vi "Test-DotNet-Event.vi"() -> ()   [LabVIEW 2013, in "EC1000-control.lvlib" / "SM1000-control.lvclass"]
uses:
  SM1000-control.lvclass
  EC1000_DOTNET/getBroadcastData-status.vi
  C:/Users/vangeste/Desktop/Libraries/EC1000-control/LECSession.dll
  LECSession.dll
  Device-identification.ctl
  DOTNET-settings.ctl
  Fixed-data-type.ctl
  Status-information.ctl
panel:
  out "serverList iterator":i32
  out "Status information":T1
  out "Job count":i32
  out "Job name list":string
  out "Fixed data":string
  in  "File name wo extension":string="AdminConfig"
  in  "Fixed data type":T2=10 items=["Controller Configuration"=5, "Laser Configuration"=6, "Lens Configuration"=2, "Correction Table"=13, "User Configuration"=15, "Performance Adjustments"=16, "Admin Configuration"=10]
  in  "Device index":i32
  out "piServerCount":i32
  out "Device identifiers":T3[](array[typedef])
  in  "DOTNET settings":T4={"Target IP"="128.178.146.163", "Target broadcast port"=11000, "Target communication port"=12200, "clientID"=-1, "Broadcast IP"="224.168.100.2", "Servercount"=-1, "Device IDs"=[]}
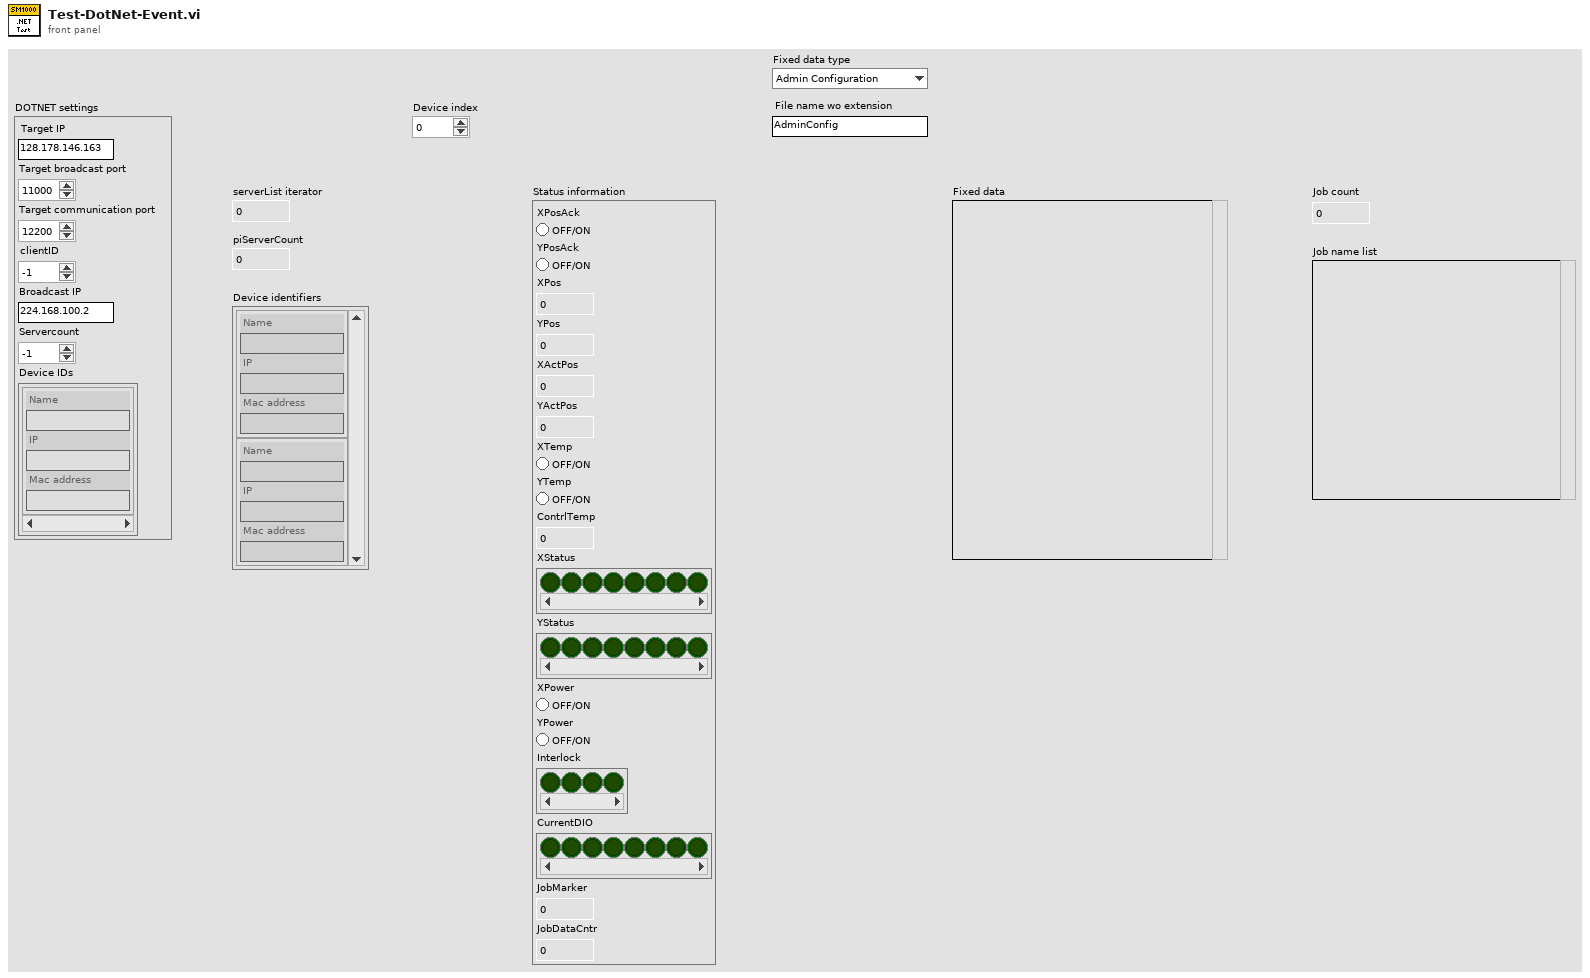
[diagram p1: front panel]
types:
  T1 = typedef "EC1000-control.lvlib/SM1000-control.lvclass/Status-information.ctl" = cluster{"XPosAck":bool, "YPosAck":bool, "XPos":i16, "YPos":i16, "XActPos":i16, "YActPos":i16, "XTemp":bool, "YTemp":bool, "ContrlTemp":i16, "XStatus":bool[], "YStatus":bool[], "XPower":bool, "YPower":bool, "Interlock":bool[], "CurrentDIO":bool[], "JobMarker":u16, "JobDataCntr":u32}
  T2 = typedef "EC1000-control.lvlib/SM1000-control.lvclass/Fixed-data-type.ctl" = i32
  T3 = typedef "EC1000-control.lvlib/SM1000-control.lvclass/Device-identification.ctl" = cluster{"Name":string, "IP":string, "Mac address":string}
  T4 = typedef "EC1000-control.lvlib/SM1000-control.lvclass/DOTNET-settings.ctl" = cluster{"Target IP":string, "Target broadcast port":i32, "Target communication port":i32, "clientID":i32, "Broadcast IP":string, "Servercount":i32, "Device IDs":T3[]}
  T5 = typedef "EC1000-control.lvlib/SM1000-control.lvclass/Object-reference.ctl" = refnum<data-value>
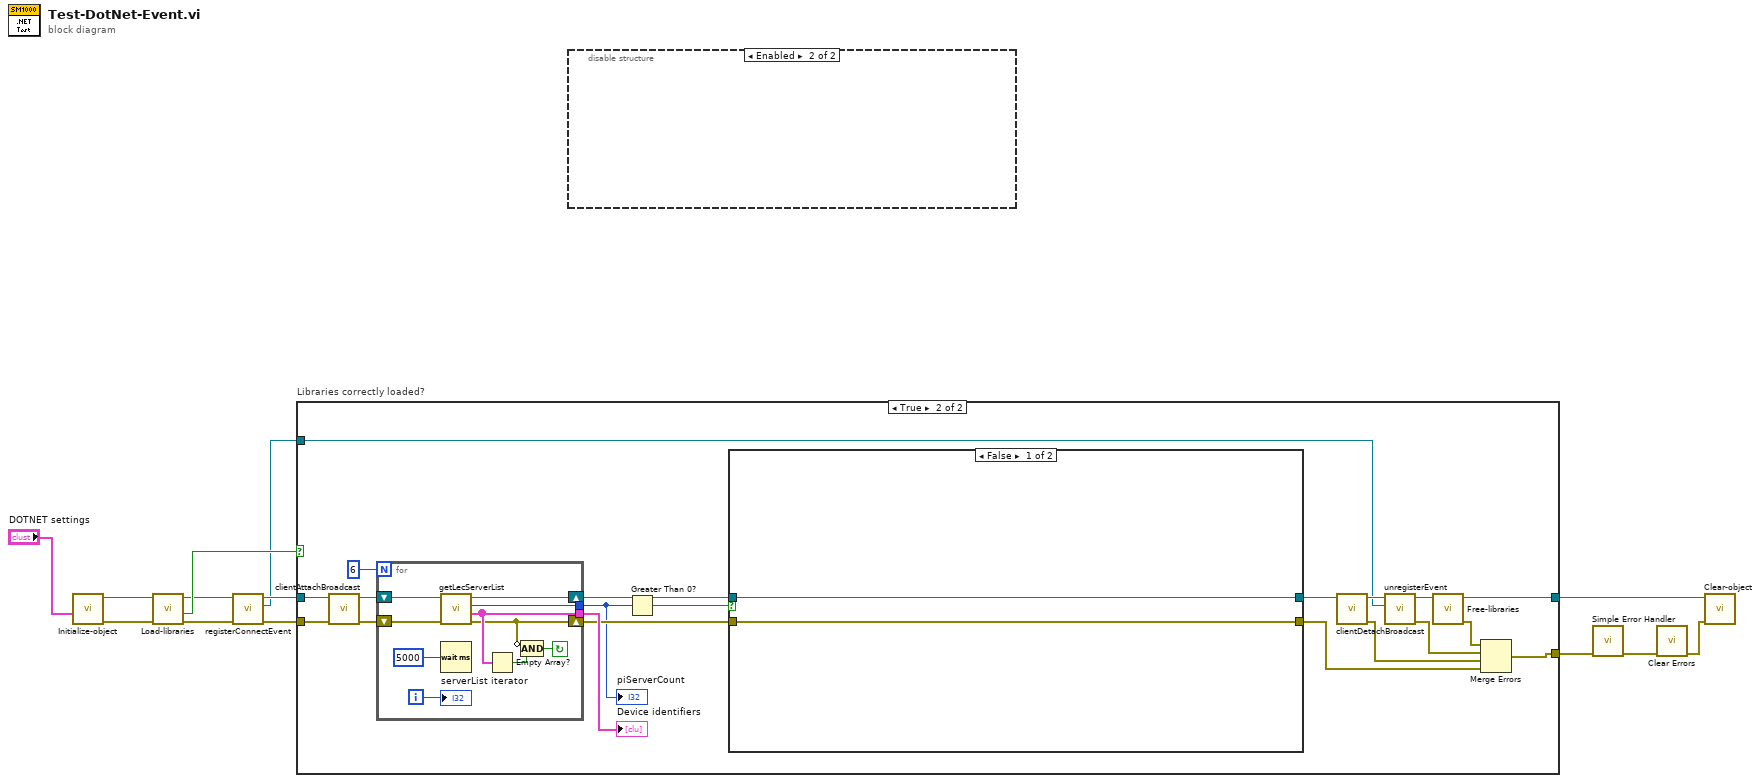
[diagram p0: block diagram]
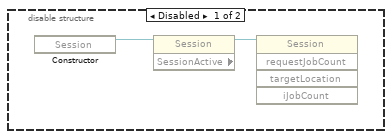
[diagram p2: hidden frame]
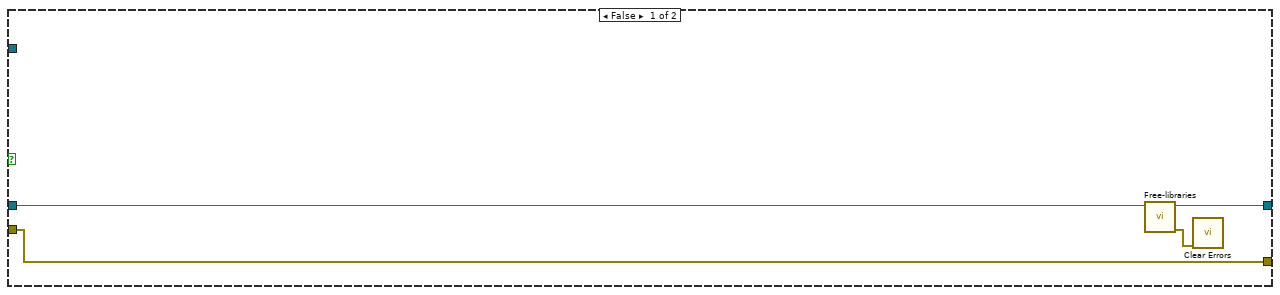
[diagram p3: hidden frame]
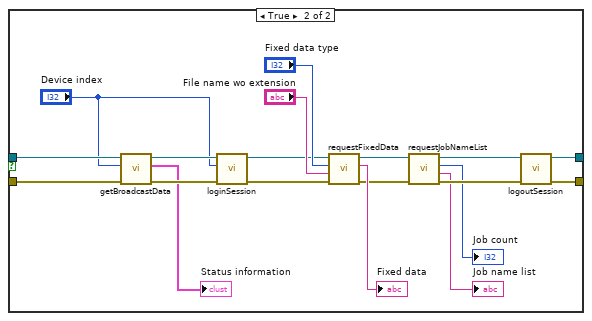
[diagram p4: hidden frame]
diagram:
  n1 = call "Initialize-object.vi"("DOTNET settings"="DOTNET settings") -> ("error out"=w11:errorcluster, "SM1000-control out"=w12:T5)  [unwired: 9 in]
  n2 = call "Load-libraries.vi"("error in (no error)"=w11, "SM1000-control in"=w12) -> ("error out"=w4:errorcluster, "Loaded?"=w10:bool, "SM1000-control out"=w5:T5)  [unwired: 7 in]
  n3 = call "registerConnectEvent.vi"("error in (no error)"=w4, "SM1000-control in"=w5) -> ("error out"=w2:errorcluster, "Event Callback"=w1:refnum<k27>, "SM1000-control out"=w3:T5)  [unwired: 7 in]
  n4 = case "Libraries correctly loaded?" shown="True" w10 {
    tunnel: w3 -> [w16 w34]
    tunnel: w2 -> [w17 w33]
    tunnel: [w17 w36] -> w8
    tunnel: [w15 w35] -> w6
    tunnel: w1 -> [_ w18]
    frame False {
      n5 = call "Free-libraries.vi"("SM1000-control in"=w16) -> ("error out"=w14:errorcluster, "SM1000-control out"=w15:T5)  [unwired: 8 in, 1 out]
      n6 = call <vilib>:"Clear Errors.vi"("error in (no error)"=w14) -> ()  [unwired: 6 in, 1 out]
    }
    frame True {
      n7 = call "clientAttachBroadcast.vi"("error in (no error)"=w33, "SM1000-control in"=w34) -> ("error out"=w30:errorcluster, "SM1000-control out"=w31:T5)  [unwired: 7 in, 1 out]
      n8 = for {
        N: 6 -> [_]
        tunnel: [w63] -> w29
        tunnel: [w66] -> w23
        shift-right: [w65] -> w25
        shift-left: w31 -> [w68]
        shift-right: [w60] -> w24
        shift-left: w30 -> [w67]
        i -> [w62]
        stop <- w59 continue-if-true
        n9 = call "getLecServerList.vi"("error in (no error)"=w67, "SM1000-control in"=w68) -> ("error out"=w60:errorcluster, "Device identifiers"=w63:T3[], "piServerCount"=w66:i32, "SM1000-control out"=w65:T5)  [unwired: 6 in]
        n10 = Wait (ms)(milliseconds to wait=u32 5000) -> ()  [unwired: 1 out]
        n11 = Empty Array?(array=w63) -> (empty?=w61:bool)
        n12 = Compound Arithmetic op=AND(invert w60, w61) -> (w59:bool)
        "serverList iterator" <- w62
      }
      "Device identifiers" <- w29
      "piServerCount" <- w23
      n13 = Greater Than 0?(x=w23) -> (x > 0?=w22:bool)
      n14 = case shown="False" w22 {
        tunnel: [w38 w58] -> w27
        tunnel: [w39 w57] -> w26
        tunnel: w25 -> [w39 w45]
        tunnel: w24 -> [w38 w44]
        frame False {
        }
        frame True {
          n15 = call-poly "getBroadcastData.vi"("error in (no error)"=w44, "Device index"="Device index", "SM1000-control in"=w45) -> ("error out"=w42:errorcluster, "Status information"=→"Status information":T1, "SM1000-control out"=w43:T5)  [unwired: 6 in]
          n16 = call "loginSession.vi"("error in (no error)"=w42, "Device index"="Device index", "SM1000-control in"=w43) -> ("error out"=w53:errorcluster, "SM1000-control out"=w54:T5)  [unwired: 7 in]
          n17 = call "requestFixedData.vi"("error in (no error)"=w53, "File name wo extension"="File name wo extension", "Fixed data type"="Fixed data type", "SM1000-control in"=w54) -> ("error out"=w50:errorcluster, "File contents"=→"Fixed data":string, "SM1000-control out"=w51:T5)  [unwired: 5 in]
          n18 = call "requestJobNameList.vi"("error in (no error)"=w50, "SM1000-control in"=w51) -> ("error out"=w48:errorcluster, "Job name list"=→"Job name list":string, "Job count"=→"Job count":i32, "SM1000-control out"=w49:T5)  [unwired: 6 in]
          n19 = call "logoutSession.vi"("error in (no error)"=w48, "SM1000-control in"=w49) -> ("error out"=w58:errorcluster, "SM1000-control out"=w57:T5)  [unwired: 8 in]
        }
      }
      n20 = call "clientDetachBroadcast.vi"("SM1000-control in"=w26) -> ("error out"=w32:errorcluster, "SM1000-control out"=w21:T5)  [unwired: 9 in]
      n21 = call "unregisterEvent.vi"("Event Callback in"=w18, "SM1000-control in"=w21) -> ("error out"=w19:errorcluster, "SM1000-control out"=w20:T5)  [unwired: 8 in]
      n22 = call "Free-libraries.vi"("SM1000-control in"=w20) -> ("error out"=w37:errorcluster, "SM1000-control out"=w35:T5)  [unwired: 8 in, 1 out]
      n23 = Merge Errors(w37, w19, w32, w27) -> (w36:errorcluster)
    }
  }
  n24 = disable-structure shown="Enabled" {
    frame Disabled {
      n25 = constructor class="Session"() -> (reference out=w70:refnum<k24>)  [unwired: 3 in, 2 out]
      n26 = property class="Session" props=["SessionActive"](reference=w70) -> (reference out=w69:refnum<k24>)  [unwired: 1 in, 2 out]
      n27 = invoke class="Session" method="requestJobCount"(reference=w69) -> ()  [unwired: 4 in, 5 out]
    }
    frame Enabled {
    }
  }
  n28 = call <vilib>:"Simple Error Handler.vi"("error in (no error)"=w8) -> ("error out"=w9:errorcluster)  [unwired: 4 in, 4 out]
  n29 = call <vilib>:"Clear Errors.vi"("error in (no error)"=w9) -> ("error out"=w7:errorcluster)  [unwired: 6 in]
  n30 = call "Clear-object.vi"("error in (no error)"=w7, "SM1000-control"=w6) -> ()  [unwired: 8 in, 2 out]
